vi "Simple Run.vi"() -> ()   [LabVIEW 2017, in "Piezo Controller.lvlib"]
uses:
  Piezo Controller.lvlib
panel:
  in  "stop":bool
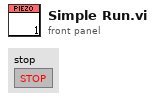
[diagram p1: front panel]
types:
  T1 = typedef "Piezo Controller.lvlib/FPGA Refs.ctl" = cluster{"FPGA VI Reference":refnum<k20>, "Instruction Target":refnum<class "niInstr FIFO Register Bus v1 Host.lvclass">, "Context":refnum<class "niInstr Instruction Framework Context v1 Host.lvclass">}
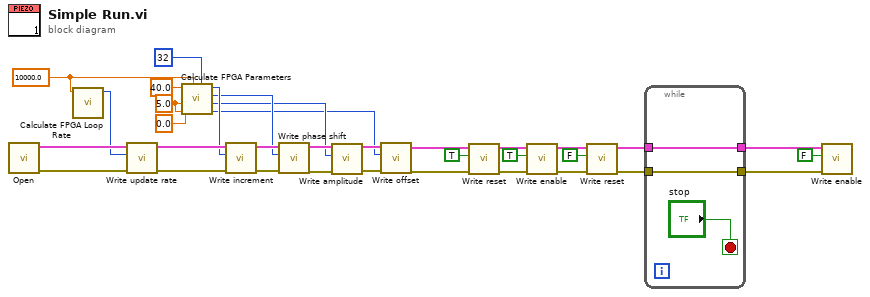
[diagram p0: block diagram]
diagram:
  w27 = 5.0 ("Signal Amplitude (V)")
  w29 = 10000.0 ("Loop Frequency (Hz)")
  n1 = call "Open.vi"() -> ("error out"=w33:errorcluster, "FPGA Refs"=w34:T1)  [unwired: 10 in]
  n2 = call "Calculate FPGA Loop Rate.vi"("Loop Frequency (Hz)"=w29) -> ("Loop  Rate (ticks)"=w32:u32)  [unwired: 10 in]
  n3 = call "Write update rate.vi"("error in (no error)"=w33, "Loop  Rate (ticks)"=w32, "FPGA Refs in"=w34) -> ("error out"=w31:errorcluster, "FPGA Refs out"=w30:T1)  [unwired: 7 in]
  n4 = call "Calculate FPGA Parameters.vi"("Accumulator Size (bit)"=32, "Loop Rate (Hz)"=w29, "Signal Offset (V)"=w27, "Signal Amplitude (V)"=w27, "Phase Shift (Deg)"=0.0, "DDS Signal Frequency (Hz)"=40.0) -> ("AO Offset"=w17:i16, "AO Amplitude"=w20:u16, "Phase Shift"=w24:u32, "Accumulator Increment"=w26:u32)  [unwired: 1 in, 1 out]
  n5 = call "Write increment.vi"("error in (no error)"=w31, "Increment"=w26, "FPGA Refs in"=w30) -> ("error out"=w23:errorcluster, "FPGA Refs out"=w25:T1)  [unwired: 7 in]
  n6 = call "Write phase shift.vi"("error in (no error)"=w23, "Phase shift"=w24, "FPGA Refs in"=w25) -> ("error out"=w22:errorcluster, "FPGA Refs out"=w21:T1)  [unwired: 7 in]
  n7 = call "Write amplitude.vi"("error in (no error)"=w22, "Amplitude"=w20, "FPGA Refs in"=w21) -> ("error out"=w19:errorcluster, "FPGA Refs out"=w18:T1)  [unwired: 7 in]
  n8 = call "Write offset.vi"("error in (no error)"=w19, "Offset"=w17, "FPGA Refs in"=w18) -> ("error out"=w15:errorcluster, "FPGA Refs out"=w16:T1)  [unwired: 7 in]
  n9 = call "Write reset.vi"("error in (no error)"=w15, "Enable"=TRUE, "FPGA Refs in"=w16) -> ("error out"=w13:errorcluster, "FPGA Refs out"=w12:T1)  [unwired: 7 in]
  n10 = call "Write enable.vi"("error in (no error)"=w13, "Enable"=TRUE, "FPGA Refs in"=w12) -> ("error out"=w10:errorcluster, "FPGA Refs out"=w9:T1)  [unwired: 7 in]
  n11 = call "Write reset.vi"("error in (no error)"=w10, "Enable"=FALSE, "FPGA Refs in"=w9) -> ("error out"=w7:errorcluster, "FPGA Refs out"=w3:T1)  [unwired: 7 in]
  n12 = while {
    tunnel: w7 -> [w36]
    tunnel: [w36] -> w5
    tunnel: [w35] -> w4
    tunnel: w3 -> [w35]
    stop <- "stop" stop-if-true
  }
  n13 = call "Write enable.vi"("error in (no error)"=w5, "Enable"=FALSE, "FPGA Refs in"=w4) -> ()  [unwired: 7 in, 2 out]
